vi "ALTS-2015 Directory Check.vi"(8 "error in (no error)":errorcluster, 11 "directory path":path) -> (0 "error out":errorcluster, 2 "exists?":bool, 3 "dup directory path":path)   [LabVIEW 2013]
doc: "Check whether a specified directory exists or not in the specified path"
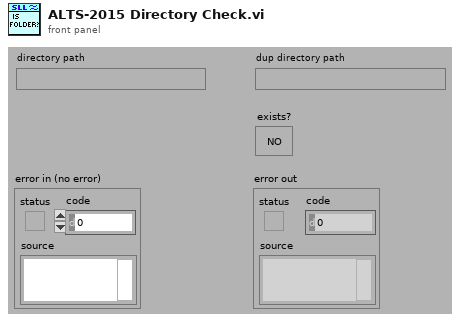
[diagram p1: front panel]
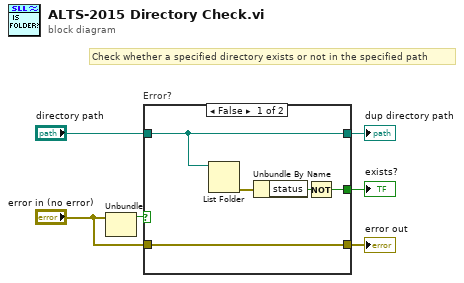
[diagram p0: block diagram]
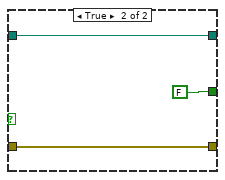
[diagram p2: hidden frame]
diagram:
  # "Check whether a specified directory exists or not in the specified path"
  n1 = Unbundle("error in (no error)") -> ("status"=w3:bool)  [unwired: 2 out]
  n2 = case "Error?" shown="False" w3 {
    tunnel: [w11 FALSE] -> w6
    tunnel: [w8 w14] -> w5
    tunnel: "directory path" -> [w8 w14]
    tunnel: [w7 w12] -> w1
    tunnel: "error in (no error)" -> [w7 w12]
    frame False {
      n3 = List Folder(path=w8) -> (error out=w10:errorcluster)  [unwired: 3 in, 3 out]
      n4 = Unbundle By Name(w10) -> ("status"=w9:bool)
      n5 = Not(x=w9) -> (.not. x?=w11:bool)
    }
    frame True {
    }
  }
  "dup directory path" <- w5
  "exists?" <- w6
  "error out" <- w1
